vi "TEST_ASIC_MAJnADDS_(4TH).vi"(4 "Serial Number":string, 5 "threshold":i32[][](array[numeric]), 6 "error in":errorcluster={"status"=FALSE, "code"=0, "source"="VISA Write in Test2_3a_ASIC_fast.vi->test_sum_ASIC.vi"}, 9 "Instrument VISA in":T1={"AWG VISA"="generadorpulsos", "Oscilloscope  VISA "="Oscilloscope", "Integration Board IP"="172.16.7.43", "connection ID"=refnum, "report out"=refnum, "report file path"=path "C:/Documents and Settings/CTA_LAB01/Desktop/L0_Asic/L0 Asic Test "}) -> (0 "error out":errorcluster, 3 "Instrument VISA out":T1={"AWG VISA"="generadorpulsos", "Oscilloscope  VISA "="Oscilloscope", "Integration Board IP"="172.16.7.43", "connection ID"=refnum, "report out"=refnum, "report file path"=path "C:/Documents and Settings/CTA_LAB01/Desktop/L0_Asic/L0 Asic Test Data"})   [LabVIEW 2009]
uses:
  <vilib>/Utility/NIReport.llb/NI_report.lvclass
  <vilib>/Utility/NIReport.llb/HTML/NI_HTML.lvclass
panel:
  in  "channel array":i32[](array[numeric])=[0, 1, 2, 3, 4, 5, 6]
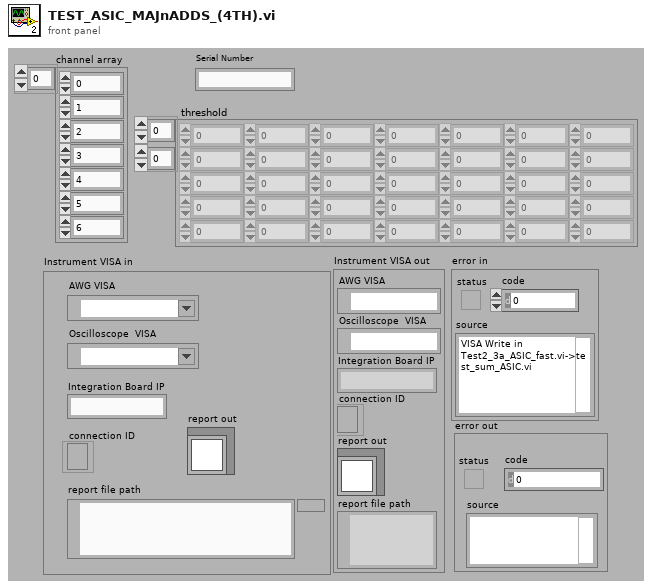
[diagram p1: front panel]
types:
  T1 = cluster{"AWG VISA":refnum<visa-resource-name>, "Oscilloscope  VISA ":refnum<visa-resource-name>, "Integration Board IP":string, "connection ID":refnum<k5>, "report out":refnum<class "NI_report.lvclass">, "report file path":path}
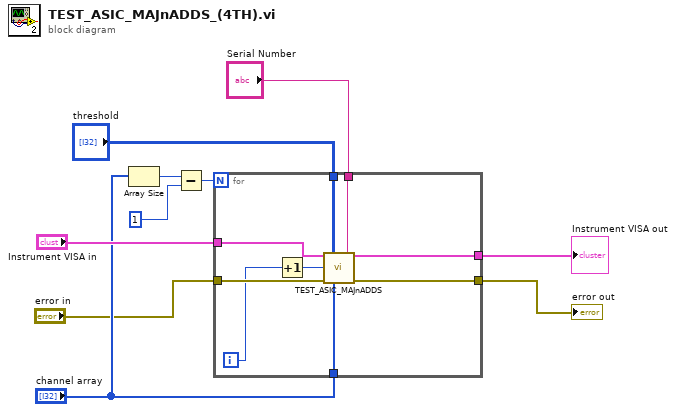
[diagram p0: block diagram]
diagram:
  n1 = Array Size(array="channel array") -> (size(s)=w5:i32)
  n2 = Subtract(x=w5, y=1) -> (x-y=w2:i32)
  n3 = for {
    N: w2 -> [_]
    tunnel: "Instrument VISA in" -> [w19]
    tunnel: "error in" -> [w18]
    tunnel: [w17] -> w9
    tunnel: [w16] -> w8
    tunnel: "channel array" -> [w15]
    tunnel: "threshold" -> [w14]
    tunnel: "Serial Number" -> [w13]
    i -> [w11]
    n4 = Increment(x=w11) -> (x+1=w12:i32)
    n5 = call "TEST_ASIC_MAJnADDS.vi"("Instrument VISA in"=w19, "threshold"=w14, "Serial number"=w13, "Cycles Burst"=w12, "error in"=w18, "channel array"=w15) -> ("Instrument VISA out"=w16:T1, "error out"=w17:errorcluster)  [unwired: 8 in]
  }
  "error out" <- w9
  "Instrument VISA out" <- w8
